vi "update action configuration.vi"(7 "action config":refnum<class "action configuration.lvclass">, 8 "error in (no error)":errorcluster, 9 "index":i32, 10 "sequence name":string, 11 "Simple Sequencer TBM configuration in":refnum<class "Simple Sequencer TBM configuration.lvclass">) -> (0 "error out":errorcluster, 3 "Simple Sequencer TBM configuration out":refnum<class "Simple Sequencer TBM configuration.lvclass">)   [LabVIEW 2015, in "Simple Sequencer TBM configuration.lvclass"]
doc: "Overwrites the action configuration at the specified sequence name and index."
uses:
  Simple Sequencer TBM configuration.lvclass
  sequencer parent classes/action configuration parent/action configuration.lvclass
  Simple Sequencer TBM configuration.lvclass/Simple Sequencer TBM configuration.ctl
  <vilib>/NI/Configuration Framework/serializable configuration/NISE_CEF_serializable configuration.lvclass
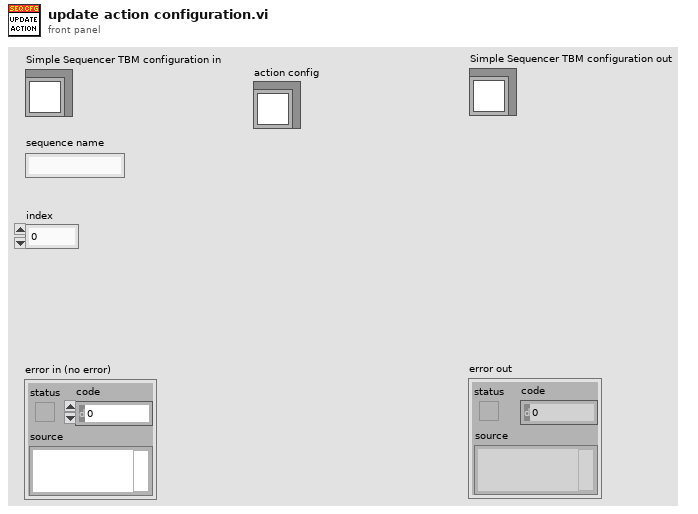
[diagram p1: front panel]
types:
  T1 = typedef "Simple Sequencer TBM configuration.lvclass/sequence definition.ctl" = cluster{"sequence name":string, "action configs":refnum<class "action configuration.lvclass">[]}
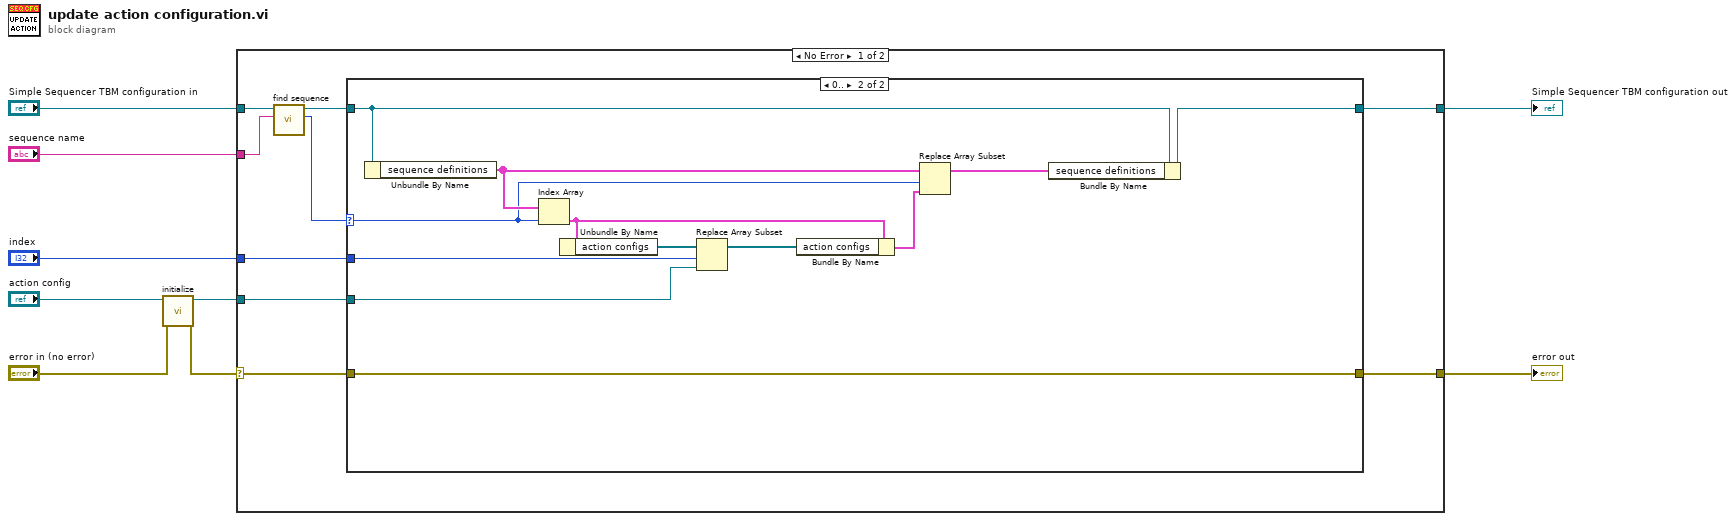
[diagram p0: block diagram]
diagram:
  n1 = call <vilib>:"initialize.vi"("error in"="error in (no error)", "configuration in"="action config") -> ("error out"=w1:errorcluster, "configuration out"=w2:refnum<class "action configuration.lvclass">)  [unwired: 7 in, 1 out]
  n2 = case shown="No Error" w1 {
    selector: w1 -> [w14 w34]
    tunnel: [w13 w34] -> w7
    tunnel: [w11 w33] -> w8
    tunnel: "Simple Sequencer TBM configuration in" -> [w18 w33]
    tunnel: "sequence name" -> [w16 _]
    tunnel: "index" -> [w12 _]
    tunnel: w2 -> [w10 _]
    frame No Error {
      n3 = call "find sequence.vi"("sequence name"=w16, "Simple Sequencer TBM configuration in"=w18) -> ("index"=w15:i32, "Simple Sequencer TBM configuration out"=w17:refnum<class "Simple Sequencer TBM configuration.lvclass">)  [unwired: 8 in]
      n4 = case shown="0.." w15 {
        selector: w15 -> [_ w28]
        tunnel: w17 -> [w19 w26]
        tunnel: w14 -> [w20 w23]
        tunnel: [w20 w23] -> w13
        tunnel: w12 -> [_ w22]
        tunnel: [w19 w24] -> w11
        tunnel: w10 -> [_ w21]
        frame ..-1 {
          # "#todo throw not found error"
        }
        frame 0.. {
          n5 = Unbundle By Name(w26) -> ("sequence definitions"=w29:T1[])
          n6 = Index Array(array=w29, index=w28) -> (element=w31:T1)
          n7 = Unbundle By Name(w31) -> ("action configs"=w32:refnum<class "action configuration.lvclass">[])
          n8 = Replace Array Subset(array=w32, new element=w21, index=w22) -> (w30:refnum<class "action configuration.lvclass">[])
          n9 = Bundle By Name(cluster=w31, "action configs"=w30) -> (w27:T1)
          n10 = Replace Array Subset(array=w29, new element=w27, index=w28) -> (w25:T1[])
          n11 = Bundle By Name(cluster=w26, "sequence definitions"=w25) -> (w24:refnum<class "Simple Sequencer TBM configuration.lvclass">)
        }
      }
    }
    frame Error {
    }
  }
  "error out" <- w7
  "Simple Sequencer TBM configuration out" <- w8
